vi "CreateAllMessageQueues.vi"(8 "entrée d'erreur":errorcluster caption="entrée d'erreur (pas d'erreur)") -> (0 "error out":errorcluster, 3 "All Message Queue Cluster":T1)   [LabVIEW 2013, in "MessageQueues.lvlib"]
doc: "Ce VI crée et nomme les piles qui seront utilisées par le programme principale. Chaque pile correspond à un appareil ou un service (sous programme).\n\nentrée :\n-error : erreur d'entrée\n\nsortie :\n- All Message Queue cluster : cluster contenant toutes les piles utilisé par le programme principale.\n- error : erreur de sortie.\n\nCe VI contruit un cluster qui englobe toutes les entité \"queues\" qui seront utilisées par le VI principale\nIl est possible d'en rajouter en copiant le ligne \"obtain Queue.vi\" et \"AddMessage.vi\"\n\nLa dénomination des queues ce fait en modifiant le cluster \"All Message Queue cluster\" \ndepuis l'objet commande stric \"All message Queue cluster.ctl\""
uses:
  MessageQueues.lvlib
  AllMessageQueue Cluster.ctl
  Message Cluster.ctl
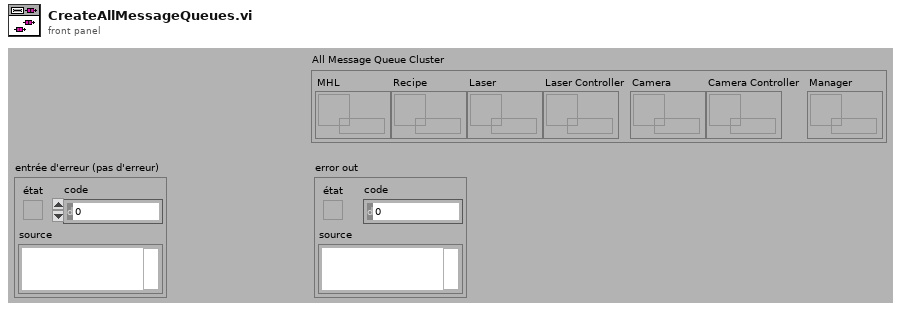
[diagram p1: front panel]
types:
  T1 = typedef "MessageQueues.lvlib/AllMessageQueue Cluster.ctl" = cluster{"MHL":refnum<queue>, "Recipe":refnum<queue>, "Laser":refnum<queue>, "Laser Controller":refnum<queue>, "Camera":refnum<queue>, "Camera Controller":refnum<queue>, "Manager":refnum<queue>}
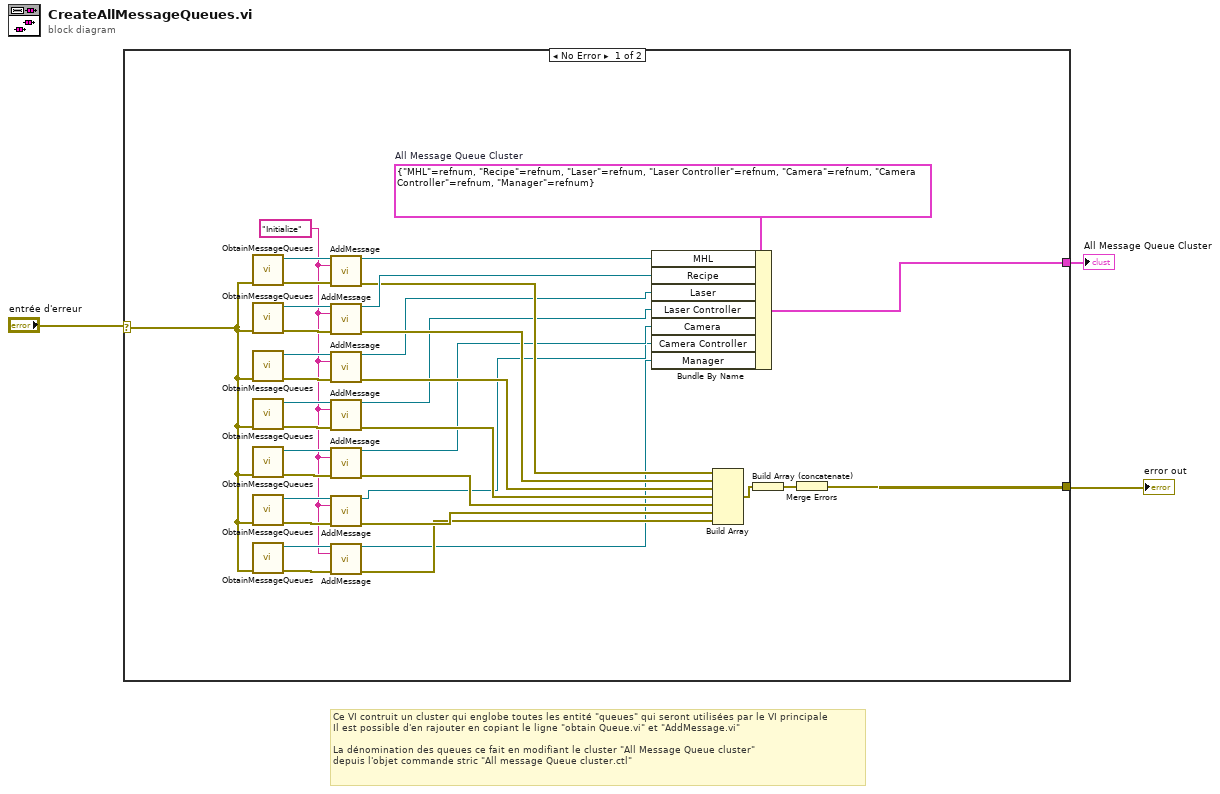
[diagram p0: block diagram]
diagram:
  # "Ce VI contruit un cluster qui englobe toutes les entité \"queues\" qui seront utilisées par le VI principale\nIl est possible d'en rajouter en copiant le ligne \"obtain Queue.vi\" et \"AddMessage.vi\"\n\nLa dénomination des queues ce fait en modifiant le cluster \"All Message Queue cluster\" \ndepuis l'objet commande stric \"All message Queue cluster.ctl\""
  n1 = case shown="No Error" "entrée d'erreur" {
    selector: "entrée d'erreur" -> [w10 w39]
    tunnel: [w29 w39] -> w2
    tunnel: [w28 _] -> w1
    frame No Error {
      w27 = T1 {"MHL"=refnum, "Recipe"=refnum, "Laser"=refnum, "Laser Controller"=refnum, "Camera"=refnum, "Camera Controller"=refnum, "Manager"=refnum}  # All Message Queue Cluster
      w9 = "Initialize"
      n2 = call "ObtainMessageQueues.vi"("entrée d'erreur (pas d'erreur)"=w10) -> ("sortie d'erreur"=w37:errorcluster, "Message queue"=w36:refnum<queue>)  [unwired: 9 in]
      n3 = call "ObtainMessageQueues.vi"("entrée d'erreur (pas d'erreur)"=w10) -> ("sortie d'erreur"=w38:errorcluster, "Message queue"=w35:refnum<queue>)  [unwired: 9 in]
      n4 = call "ObtainMessageQueues.vi"("entrée d'erreur (pas d'erreur)"=w10) -> ("sortie d'erreur"=w26:errorcluster, "Message queue"=w24:refnum<queue>)  [unwired: 9 in]
      n5 = call "ObtainMessageQueues.vi"("entrée d'erreur (pas d'erreur)"=w10) -> ("sortie d'erreur"=w25:errorcluster, "Message queue"=w23:refnum<queue>)  [unwired: 9 in]
      n6 = call "ObtainMessageQueues.vi"("entrée d'erreur (pas d'erreur)"=w10) -> ("sortie d'erreur"=w18:errorcluster, "Message queue"=w19:refnum<queue>)  [unwired: 9 in]
      n7 = call "ObtainMessageQueues.vi"("entrée d'erreur (pas d'erreur)"=w10) -> ("sortie d'erreur"=w17:errorcluster, "Message queue"=w16:refnum<queue>)  [unwired: 9 in]
      n8 = call "ObtainMessageQueues.vi"("entrée d'erreur (pas d'erreur)"=w10) -> ("sortie d'erreur"=w12:errorcluster, "Message queue"=w13:refnum<queue>)  [unwired: 9 in]
      n9 = call "AddMessage.vi"("Message queue"=w36, "Message"=w9, "entrée d'erreur (pas d'erreur)"=w37) -> ("Dup Message queue"=w33:refnum<queue>, "error out"=w32:errorcluster)  [unwired: 11 in]
      n10 = call "AddMessage.vi"("Message queue"=w35, "Message"=w9, "entrée d'erreur (pas d'erreur)"=w38) -> ("Dup Message queue"=w34:refnum<queue>, "error out"=w31:errorcluster)  [unwired: 11 in]
      n11 = call "AddMessage.vi"("Message queue"=w24, "Message"=w9, "entrée d'erreur (pas d'erreur)"=w26) -> ("Dup Message queue"=w8:refnum<queue>, "error out"=w22:errorcluster)  [unwired: 11 in]
      n12 = call "AddMessage.vi"("Message queue"=w23, "Message"=w9, "entrée d'erreur (pas d'erreur)"=w25) -> ("Dup Message queue"=w7:refnum<queue>, "error out"=w21:errorcluster)  [unwired: 11 in]
      n13 = call "AddMessage.vi"("Message queue"=w19, "Message"=w9, "entrée d'erreur (pas d'erreur)"=w18) -> ("Dup Message queue"=w6:refnum<queue>, "error out"=w14:errorcluster)  [unwired: 11 in]
      n14 = call "AddMessage.vi"("Message queue"=w16, "Message"=w9, "entrée d'erreur (pas d'erreur)"=w17) -> ("Dup Message queue"=w5:refnum<queue>, "error out"=w15:errorcluster)  [unwired: 11 in]
      n15 = call "AddMessage.vi"("Message queue"=w13, "Message"=w9, "entrée d'erreur (pas d'erreur)"=w12) -> ("Dup Message queue"=w4:refnum<queue>, "error out"=w11:errorcluster)  [unwired: 11 in]
      n16 = Bundle By Name(cluster=w27, "MHL"=w33, "Recipe"=w34, "Laser"=w8, "Laser Controller"=w7, "Camera"=w6, "Camera Controller"=w5, "Manager"=w4) -> (w28:T1)
      n17 = Build Array(w32, w31, w22, w21, w14, w15, w11) -> (w30:errorcluster[])
      n18 = Build Array (concatenate)(w30) -> (w20:errorcluster[])
      n19 = Merge Errors(w20) -> (w29:errorcluster)
    }
    frame Error {
    }
  }
  "error out" <- w2
  "All Message Queue Cluster" <- w1
